vi "Get_CPU_Model_Name.vi"() -> (3 "CPU Model":string)   [LabVIEW 2020]
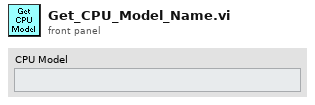
[diagram p1: front panel]
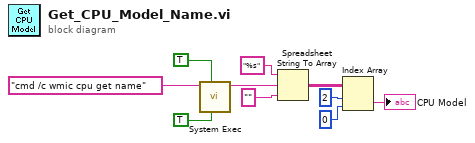
[diagram p0: block diagram]
diagram:
  n1 = call <vilib>:"System Exec.vi"("run minimized? (F)"=TRUE, "wait until completion? (T)"=TRUE, "command line"="cmd /c wmic cpu get name") -> ("standard output"=w7:string)  [unwired: 5 in, 3 out]
  n2 = Spreadsheet String To Array(format string="%s", spreadsheet string=w7, array type (2D Dbl)="" ("command line")) -> (array=w4:string[][])  [unwired: 1 in]
  n3 = Index Array(array=w4, index (row)=2 ("disabled index (row)"), index (col)=0 ("disabled index (col)")) -> (element=→"CPU Model":string)
